vi "setState.vi"(8 "error in (no error)":errorcluster, 9 "state":cluster{"state_name":string, "value":string}, 10 "index":i32, 11 "Channel.lvclass in":refnum<class "Channel.lvclass">) -> (0 "error out":errorcluster, 3 "Channel.lvclass out":refnum<class "Channel.lvclass">)   [LabVIEW 2009, in "Tools.lvlib" / "DatabaseHelpers.lvlib" / "Channel.lvclass"]
uses:
  Channel.lvclass
  Channel.lvclass/Channel.ctl
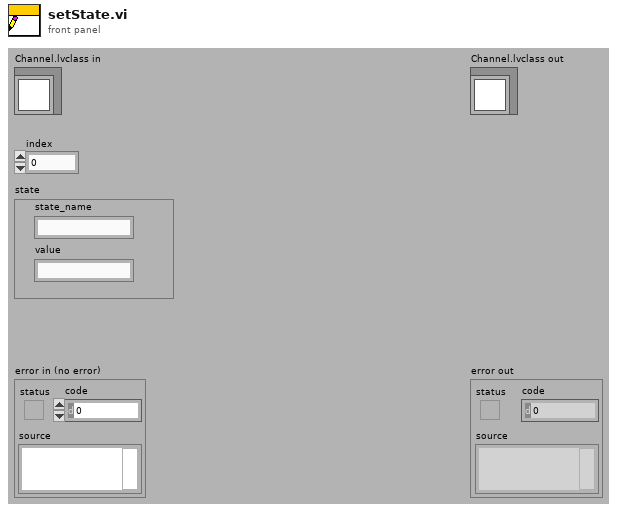
[diagram p1: front panel]
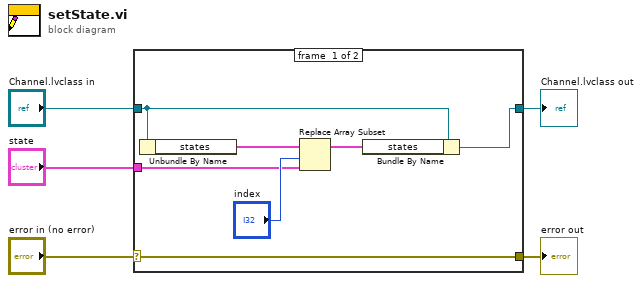
[diagram p0: block diagram]
diagram:
  n1 = case shown="No Error" "error in (no error)" {
    selector: "error in (no error)" -> [w12 w13]
    tunnel: [w12 w13] -> w4
    tunnel: [w11 w14] -> w2
    tunnel: "Channel.lvclass in" -> [w10 w14]
    tunnel: "state" -> [w6 _]
    frame #0 {
      n2 = Unbundle By Name(w10) -> ("states"=w9:cluster{"state_name":string, "value":string}[])
      n3 = Replace Array Subset(array=w9, new element=w6, index="index") -> (w8:cluster{"state_name":string, "value":string}[])
      n4 = Bundle By Name(cluster=w10, "states"=w8) -> (w11:refnum<class "Channel.lvclass">)
    }
    frame #1 {
    }
  }
  "error out" <- w4
  "Channel.lvclass out" <- w2
